vi "到期.vi"(2 "最终选择的真实的日期":dbl[](array[numeric]), 3 "加期限后的日期":dbl[](array[numeric]), 4 "密码和期限":string[][](array[string]), 5 "密码输入":string) -> (0 "密码生效":bool, 1 "到期了":bool)   [LabVIEW 2016]
uses:
  <vilib>/Utility/file.llb/Write Delimited Spreadsheet (DBL).vi
  <vilib>/Utility/file.llb/Write Delimited Spreadsheet (string).vi
panel:
  out "密码":string[](array[string])
  out "期限（月）":string[](array[string])
  out "密码":string[](array[string])
  out "比较的日期":dbl
  out "当前日期":u32
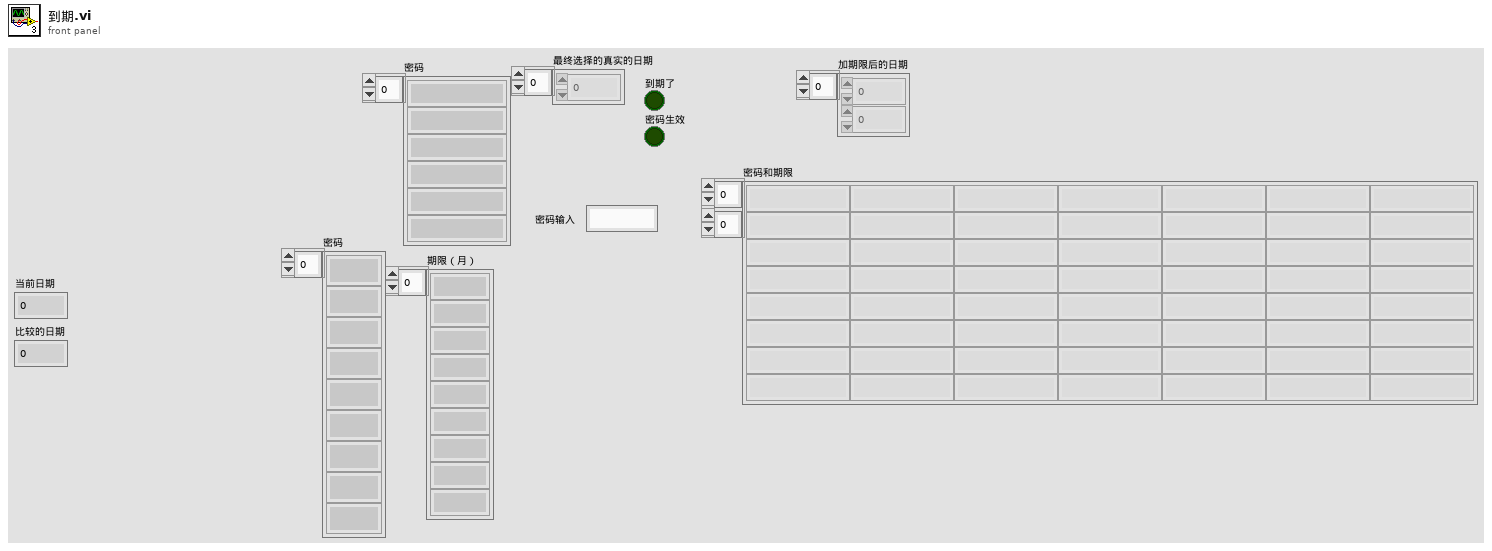
[diagram p1: front panel]
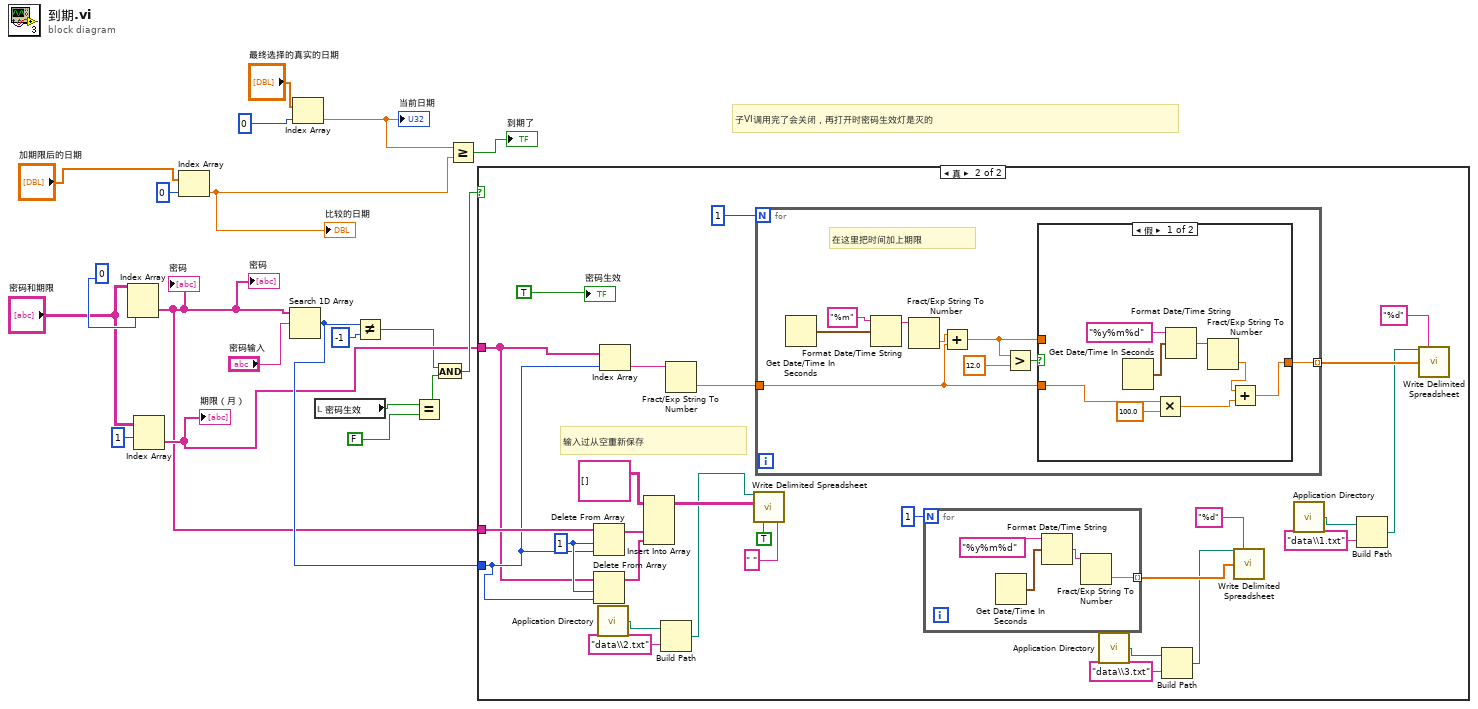
[diagram p0: block diagram]
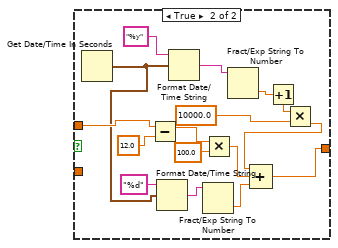
[diagram p3: hidden frame]
diagram:
  # "子VI调用完了会关闭，再打开时密码生效灯是灭的"
  n1 = Index Array(array="密码和期限", index (row)=0 ("索引 (行)")) -> (element=w7:string[])  [unwired: 1 in]
  "密码" <- w7
  "密码" <- w7
  n2 = Index Array(array="密码和期限", index (row)=1 ("索引 (行)")) -> (element=w9:string[])  [unwired: 1 in]
  "期限（月）" <- w9
  n3 = Index Array(array="加期限后的日期", index=0 ("索引")) -> (element=w11:dbl)
  "比较的日期" <- w11
  n4 = Search 1D Array(1D array=w7, element="密码输入") -> (index of element=w14:i32)  [unwired: 1 in]
  n5 = Index Array(array="最终选择的真实的日期", index=0 ("索引")) -> (element=w3:dbl)
  "当前日期" <- w3
  n6 = local read "密码生效"() -> (w19:bool)
  n7 = Not Equal?(x=w14, y=-1) -> (x != y?=w4:bool)
  n8 = Equal?(x=w19, y=FALSE) -> (x = y?=w16:bool)
  n9 = And(x=w4, y=w16) -> (x .and. y?=w17:bool)
  n10 = Greater Or Equal?(x=w3, y=w11) -> (x >= y?=→"到期了":bool)
  n11 = case shown="真" w17 {
    tunnel: w14 -> [_ w43]
    tunnel: w7 -> [_ w46]
    tunnel: w9 -> [_ w34]
    frame False {
    }
    frame True {
      w44 = 1 ("索引")
      # "输入过从空重新保存"
      n12 = Delete From Array(array=w46, length=w44, index=w43) -> (array with subset deleted=w41:string[])  [unwired: 1 out]
      n13 = Delete From Array(array=w34, length=w44, index=w43) -> (array with subset deleted=w40:string[])  [unwired: 1 out]
      n14 = call <vilib>:"Application Directory.vi"() -> ("Application Directory"=w29:path)
      n15 = Index Array(array=w34, index=w43) -> (element=w38:string)
      n16 = Insert Into Array(array=string[][] [] ("数组"), new element #1=w41, new element #2=w40) -> (w39:string[][])  [unwired: 2 in]
      n17 = Build Path(base path=w29, name or relative path="data\\2.txt" ("名称或相对路径")) -> (appended path=w27:path)
      n18 = Fract/Exp String To Number(string=w38) -> (number=w37:dbl)  [unwired: 3 in, 1 out]
      n19 = call-poly <vilib>:"Write Delimited Spreadsheet.vi"("file path (dialog if empty)"=w27, "2D data"=w39, "transpose? (no:F)"=TRUE, "delimiter (\\t)"=" " ("delimiter (\\t)")) -> ()  [unwired: 10 in, 2 out]
      n20 = for {
        N: 1 -> [_]
        tunnel: w37 -> [w55]
        tunnel: [w54] -> w35 mode=indexing
        # "在这里把时间加上期限"
        n21 = Get Date/Time In Seconds() -> (seconds since 1Jan1904=w61:timestamp)
        n22 = Format Date/Time String(time format string (%c)="%m" ("时间格式字符串(%c)"), seconds (now)=w61) -> (date/time string=w58:string)  [unwired: 1 in]
        n23 = Fract/Exp String To Number(string=w58) -> (number=w59:dbl)  [unwired: 3 in, 1 out]
        n24 = Add(x=w59, y=w55) -> (x+y=w53:dbl)
        n25 = Greater?(x=w53, y=12.0) -> (0:w56:bool)
        n26 = case shown="假" w56 {
          tunnel: w55 -> [w66 _]
          tunnel: [w62 w70] -> w54
          tunnel: w53 -> [_ w85]
          frame False {
            n27 = Get Date/Time In Seconds() -> (seconds since 1Jan1904=w68:timestamp)
            n28 = Multiply(x=w66, y=100.0) -> (x*y=w63:dbl)
            n29 = Format Date/Time String(time format string (%c)="%y%m%d" ("时间格式字符串(%c)"), seconds (now)=w68) -> (date/time string=w69:string)  [unwired: 1 in]
            n30 = Fract/Exp String To Number(string=w69) -> (number=w64:dbl)  [unwired: 3 in, 1 out]
            n31 = Add(x=w64, y=w63) -> (x+y=w62:dbl)
          }
          frame True {
            n32 = Get Date/Time In Seconds() -> (seconds since 1Jan1904=w75:timestamp)
            n33 = Subtract(x=w85, y=12.0) -> (x-y=w78:dbl)
            n34 = Format Date/Time String(time format string (%c)="%d" ("时间格式字符串(%c)"), seconds (now)=w75) -> (date/time string=w74:string)  [unwired: 1 in]
            n35 = Format Date/Time String(time format string (%c)="%y" ("时间格式字符串(%c)"), seconds (now)=w75) -> (date/time string=w82:string)  [unwired: 1 in]
            n36 = Fract/Exp String To Number(string=w74) -> (number=w73:dbl)  [unwired: 3 in, 1 out]
            n37 = Multiply(x=w78, y=100.0) -> (x*y=w72:dbl)
            n38 = Fract/Exp String To Number(string=w82) -> (number=w81:dbl)  [unwired: 3 in, 1 out]
            n39 = Increment(x=w81) -> (x+1=w80:dbl)
            n40 = Multiply(x=w80, y=10000.0) -> (x*y=w71:dbl)
            n41 = Compound Arithmetic op=ADD(w71, w72, w73) -> (w70:dbl)
          }
        }
      }
      n42 = for {
        N: 1 -> [_]
        tunnel: [w49] -> w30 mode=indexing
        n43 = Get Date/Time In Seconds() -> (seconds since 1Jan1904=w51:timestamp)
        n44 = Format Date/Time String(time format string (%c)="%y%m%d" ("时间格式字符串(%c)"), seconds (now)=w51) -> (date/time string=w50:string)  [unwired: 1 in]
        n45 = Fract/Exp String To Number(string=w50) -> (number=w49:dbl)  [unwired: 3 in, 1 out]
      }
      n46 = call <vilib>:"Application Directory.vi"() -> ("Application Directory"=w25:path)
      n47 = Build Path(base path=w25, name or relative path="data\\3.txt" ("名称或相对路径")) -> (appended path=w24:path)
      n48 = call-poly <vilib>:"Write Delimited Spreadsheet.vi"("file path (dialog if empty)"=w24, "format (%.3f)"="%d" ("format (%d)"), "1D data"=w30) -> ()  [unwired: 11 in, 2 out]
      n49 = call <vilib>:"Application Directory.vi"() -> ("Application Directory"=w23:path)
      n50 = Build Path(base path=w23, name or relative path="data\\1.txt" ("名称或相对路径")) -> (appended path=w21:path)
      n51 = call-poly <vilib>:"Write Delimited Spreadsheet.vi"("file path (dialog if empty)"=w21, "format (%.3f)"="%d" ("format (%d)"), "1D data"=w35) -> ()  [unwired: 11 in, 2 out]
      "密码生效" <- TRUE ("x >= y? 2")
    }
  }
